vi "Get Result.vi"(1 "Act_Get One.lvclass":refnum<class "Act_Get One.lvclass">) -> (0 "Result":refnum<class>)   [LabVIEW 2014, in "Act_Get One.lvclass"]
uses:
  Act_Get One.lvclass
  Act_Get One.lvclass/Act_Get One.ctl
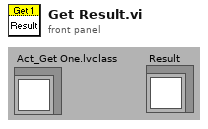
[diagram p1: front panel]
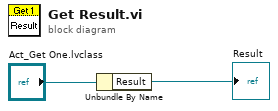
[diagram p0: block diagram]
diagram:
  n1 = Unbundle By Name("Act_Get One.lvclass") -> ("Result"=→"Result":refnum<class>)
